vi "Tab Dawn.vi"(11 "output cluster":T3) -> (3 "output cluster 2":T2)   [LabVIEW 2020, in "MDI ViewManager.lvlib"]
uses:
  MDI ViewManager.lvlib
  <vilib>/Utility/miscctls.llb/LVPoint32TypeDef.ctl
  <vilib>/Utility/cursorutil.llb/Set Cursor (Icon Pict).vi
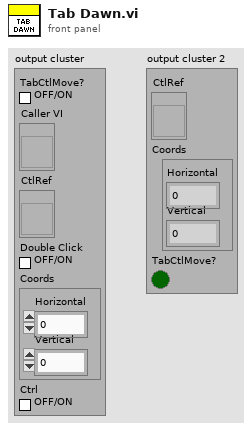
[diagram p1: front panel]
types:
  T1 = typedef "LVPoint32TypeDef.ctl" = cluster{"Horizontal":i32, "Vertical":i32}
  T2 = cluster{"CtlRef":refnum<vi>, "Coords":T1, "TabCtlMove?":bool}
  T3 = cluster{"TabCtlMove?":bool, "Caller VI":refnum<vi>, "CtlRef":refnum<vi>, "Double Click":bool, "Coords":T1, "Ctrl":bool}
  T4 = typedef "LVPositionTypeDef.ctl" = cluster{"Left":i32, "Top":i32}
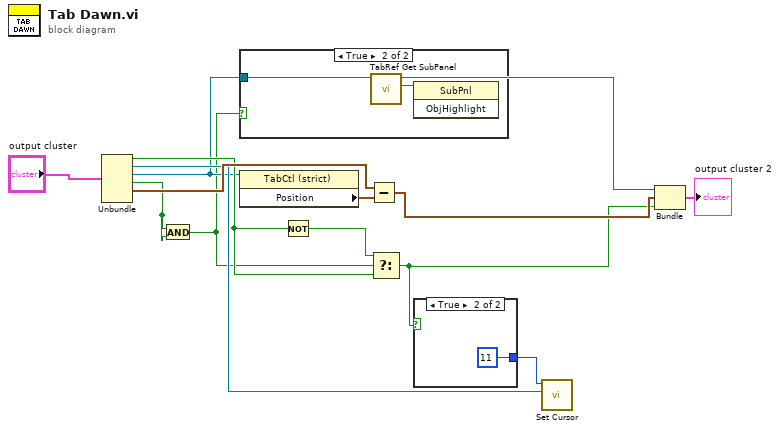
[diagram p0: block diagram]
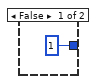
[diagram p3: hidden frame]
diagram:
  n1 = Unbundle("output cluster") -> ("TabCtlMove?"=w8:bool, "Caller VI"=w7:refnum<vi>, "CtlRef"=w6:refnum<vi>, "Double Click"=w1:bool, "Coords"=w9:T1)  [unwired: 1 out]
  n2 = And(x=w1, y=w1) -> (x .and. y?=w2:bool)
  n3 = case shown="True" w2 {
    tunnel: w6 -> [_ w14]
    frame False {
    }
    frame True {
      n4 = call "TabRef Get SubPanel.vi"("TabControl in"=w14) -> ("Sub Panel"=w15:refnum<vi>)  [unwired: 8 in, 2 out]
      n5 = invoke class="SubPnl" method="ObjHighlight"(reference=w15) -> ()  [unwired: 2 in, 3 out]
    }
  }
  n6 = property class="TabCtl (strict)"(reference=w6) -> ("Position"=w13:T4)  [unwired: 1 in, 2 out]
  n7 = Not(x=w8) -> (.not. x?=w11:bool)
  n8 = Subtract(x=w9, y=w13) -> (x-y=w5:T1)
  n9 = Select(t=w11, s=w2, f=w8) -> (s? t:f=w4:bool)
  n10 = case shown="True" w4 {
    tunnel: [u16 1 ("icon") u16 11 ("icon")] -> w12
    frame False {
    }
    frame True {
    }
  }
  n11 = call-poly <vilib>:"Set Cursor.vi"("VI reference (current VI)"=w7, "icon"=w12) -> ()  [unwired: 8 in, 2 out]
  n12 = Bundle("CtlRef"=w6, "Coords"=w5, "TabCtlMove?"=w4) -> (→"output cluster 2":T2)  [unwired: 1 in]
